vi "LEP_RV_MemoryMap_SetDefaults.vi"(0 "Config In":T1[](array[typedef]), 5 "SourceFiles":path[](array[path]), 11 "error in (no error)":errorcluster) -> (4 "Config Out":T1[](array[typedef]), 6 "Section Names":string[](array[string]), 15 "error out":errorcluster)   [LabVIEW 2011]
doc: "Define default memory mapping for the Axiom CMD565 target."
uses:
  <vilib>/LabVIEW Targets/Embedded/Utilities/MemMap/EMB_Utility_MemMap_VI_Config.ctl
  <vilib>/LabVIEW Targets/Embedded/Utilities/MemMap/EMB_Utility_MemMap_VI_Type.ctl
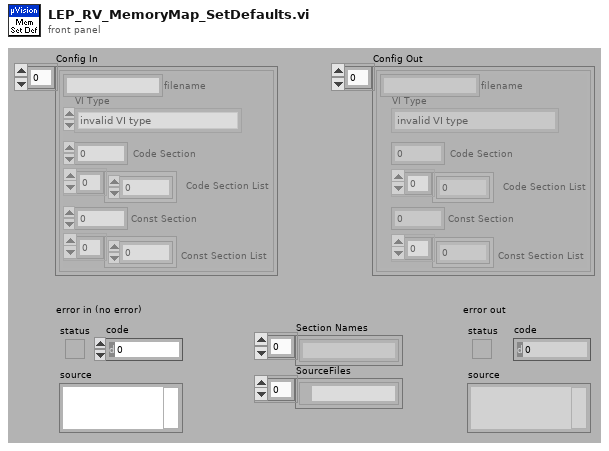
[diagram p1: front panel]
types:
  T1 = typedef "EMB_Utility_MemMap_VI_Config.ctl" = cluster{"filename":string, "Code Section":i32, "Code Section List":i32[], "Const Section":i32, "Const Section List":i32[], "VI Type":T2}
  T2 = typedef "EMB_Utility_MemMap_VI_Type.ctl" = enum32{"invalid VI type", "Standard VI", "Control VI", "Global VI", "Polymorphic VI", "Configuration VI", "SubSystem"}
  T3 = enum32{"invalid VI type", "Standard VI", "Control VI", "Global VI", "Polymorphic VI", "Configuration VI", "SubSystem", "Facade VI", "Method VI", "Statechart Diagram VI"}
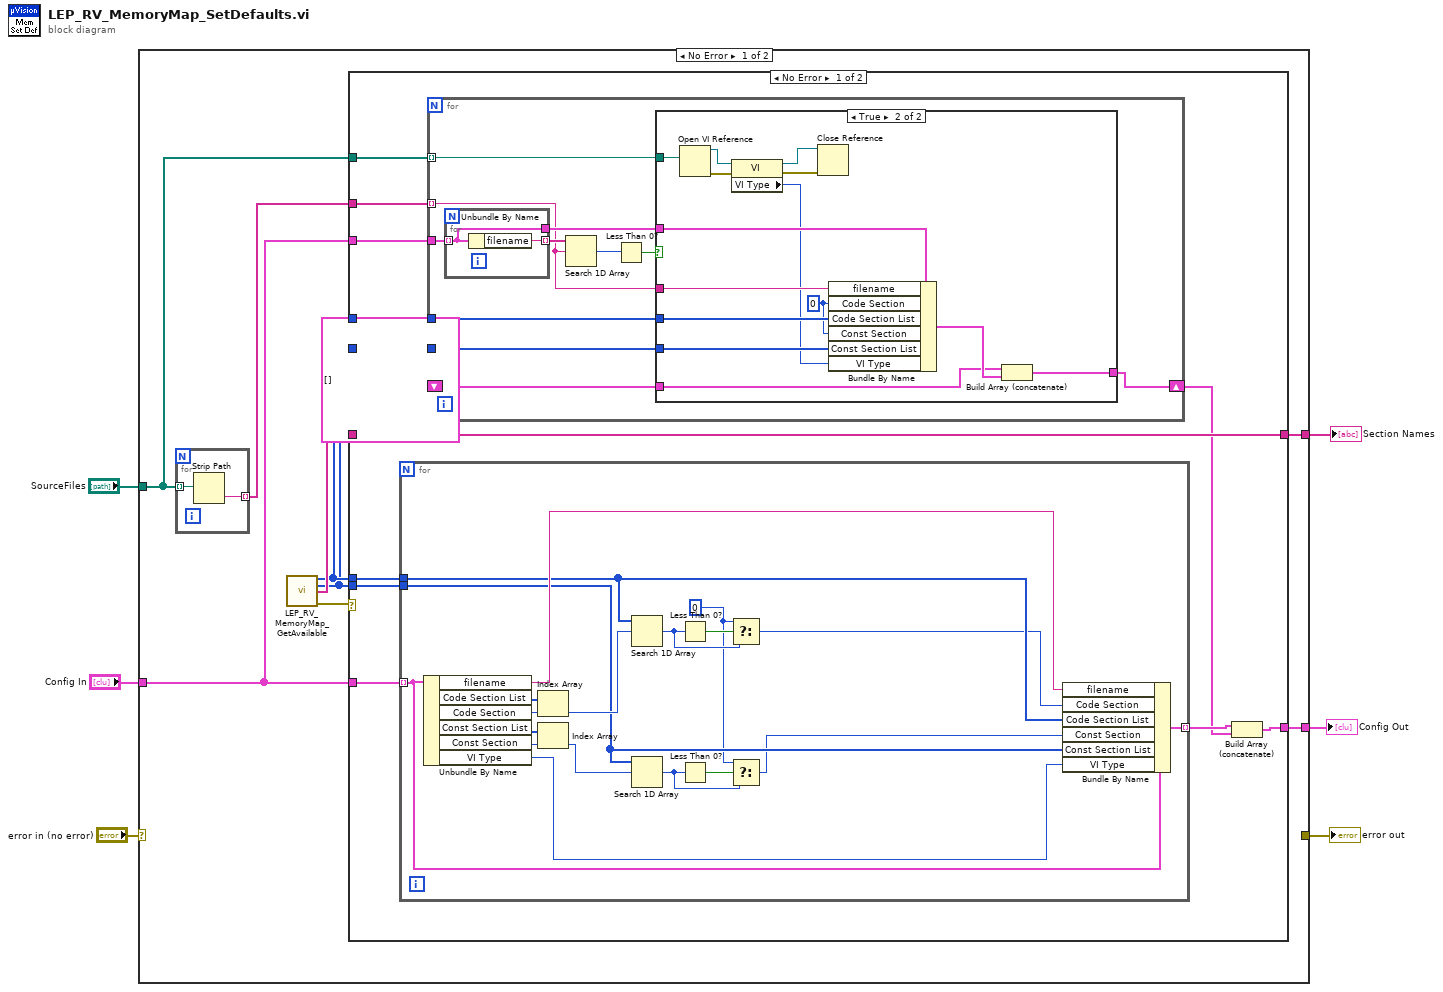
[diagram p0: block diagram]
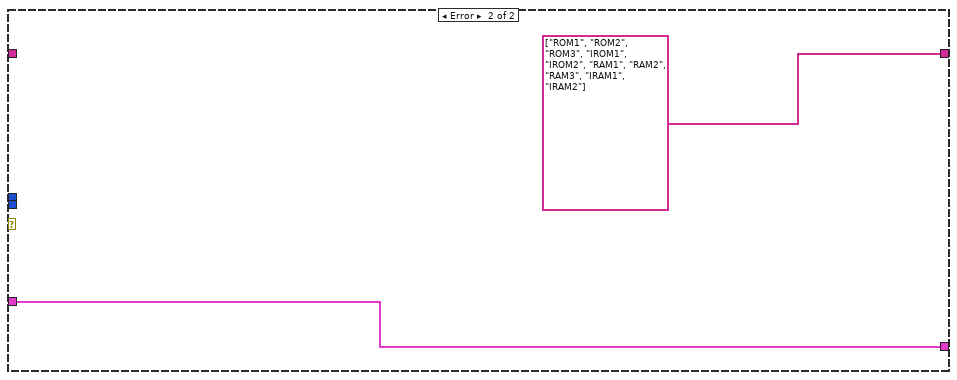
[diagram p3: hidden frame]
diagram:
  n1 = case shown="No Error" "error in (no error)" {
    selector: "error in (no error)" -> [_ w81]
    tunnel: [_ w81] -> w5
    tunnel: "Config In" -> [w10 w80]
    tunnel: [w15 w80] -> w3
    tunnel: [w12 _] -> w2
    tunnel: "SourceFiles" -> [w7 _]
    frame No Error {
      n2 = for {
        tunnel: [w17] -> w11 mode=indexing
        tunnel: w7 -> [w16] mode=indexing
        n3 = Strip Path(path=w16) -> (name=w17:string)  [unwired: 1 out]
      }
      n4 = call "LEP_RV_MemoryMap_GetAvailable.vi"() -> ("Code Section List"=w9:i32[], "Data Section List"=w8:i32[], "Section Names"=w13:string[], "error out"=w14:errorcluster)  [unwired: 10 in, 2 out]
      n5 = case shown="No Error" w14 {
        tunnel: w10 -> [w30 w79]
        tunnel: [w22 w79] -> w15
        tunnel: w9 -> [w29 _]
        tunnel: w8 -> [w28 _]
        tunnel: w13 -> [w27 _]
        tunnel: [w27 string[] ["ROM1", "ROM2", "ROM3", "IROM1", "IROM2", "RAM1", "RAM2", "RAM3", "IRAM1", "IRAM2"]] -> w12
        tunnel: w11 -> [w26 _]
        tunnel: w10 -> [w25 _]
        tunnel: w9 -> [w24 _]
        tunnel: w8 -> [w23 _]
        tunnel: w7 -> [w18 _]
        frame No Error {
          n6 = for {
            tunnel: w30 -> [w75] mode=indexing
            tunnel: [w74] -> w21 mode=indexing
            tunnel: w29 -> [w69]
            tunnel: w28 -> [w63]
            w59 = 0 ("t")
            n7 = Unbundle By Name(w75) -> ("filename"=w76:string, "Code Section List"=w71:i32[], "Code Section"=w70:i32, "Const Section List"=w73:i32[], "Const Section"=w72:i32, "VI Type"=w77:T2)
            n8 = Index Array(array=w71, index=w70) -> (element=w68:i32)
            n9 = Index Array(array=w73, index=w72) -> (element=w62:i32)
            n10 = Search 1D Array(1D array=w69, element=w68) -> (index of element=w66:i32)  [unwired: 1 in]
            n11 = Search 1D Array(1D array=w63, element=w62) -> (index of element=w64:i32)  [unwired: 1 in]
            n12 = Less Than 0?(x=w66) -> (x < 0?=w67:bool)
            n13 = Less Than 0?(x=w64) -> (x < 0?=w65:bool)
            n14 = Select(t=w59, s=w67, f=w66) -> (s? t:f=w61:i32)
            n15 = Select(t=w59, s=w65, f=w64) -> (s? t:f=w60:i32)
            n16 = Bundle By Name(cluster=w75, "filename"=w76, "Code Section"=w61, "Code Section List"=w69, "Const Section"=w60, "Const Section List"=w63, "VI Type"=w77) -> (w74:T1)
          }
          n17 = for {
            tunnel: w26 -> [w34] mode=indexing
            tunnel: w25 -> [w41]
            tunnel: w24 -> [w36]
            tunnel: w23 -> [w35]
            shift-right: [w33] -> w20
            shift-left: T1[] [] -> [w32]
            tunnel: w18 -> [w31] mode=indexing
            n18 = for {
              tunnel: w41 -> [w57] mode=indexing
              tunnel: [w58] -> w40 mode=indexing
              tunnel: [w57] -> w37
              n19 = Unbundle By Name(w57) -> ("filename"=w58:string)
            }
            n20 = Search 1D Array(1D array=w40, element=w34) -> (index of element=w39:i32)  [unwired: 1 in]
            n21 = Less Than 0?(x=w39) -> (x < 0?=w38:bool)
            n22 = case shown="True" w38 {
              tunnel: w37 -> [_ w56]
              tunnel: w36 -> [_ w55]
              tunnel: w35 -> [_ w54]
              tunnel: w34 -> [_ w53]
              tunnel: [w42 w52] -> w33
              tunnel: w32 -> [w42 w50]
              tunnel: w31 -> [_ w45]
              frame False {
              }
              frame True {
                w43 = 0 ("Code Section")
                n23 = Open VI Reference(vi path=w45) -> (vi reference=w47:refnum<vi>, error out=w49:errorcluster)  [unwired: 5 in]
                n24 = property class="VI"(reference=w47, error in=w49) -> (reference out=w46:refnum<vi>, error out=w48:errorcluster, "VI Type"=w44:T3)
                n25 = Close Reference(reference=w46, error in (no error)=w48) -> ()  [unwired: 1 out]
                n26 = Bundle By Name(cluster=w56, "filename"=w53, "Code Section"=w43, "Code Section List"=w55, "Const Section"=w43, "Const Section List"=w54, "VI Type"=w44) -> (w51:T1)
                n27 = Build Array (concatenate)(w50, w51) -> (w52:T1[])
              }
            }
          }
          n28 = Build Array (concatenate)(w21, w20) -> (w22:T1[])
        }
        frame Error {
        }
      }
    }
    frame Error {
    }
  }
  "error out" <- w5
  "Config Out" <- w3
  "Section Names" <- w2
